vi "CANOpen Addon Initialization VI.vi"(8 "error in (no error)":errorcluster, 10 "Custom XML":string, 11 "Device Item Ref in":T1 format="%.0x") -> (0 "error out":errorcluster, 3 "Device Item Ref out":T1 format="%.0x")   [LabVIEW 2013, in "CANOpen Addon Custom Device.lvlib"]
uses:
  CANOpen Addon Custom Device.lvlib
  <vilib>/NI Veristand/Custom Device API/Custom Device Item Ref.ctl
  <vilib>/NI Veristand/Custom Device API/Custom Device Channel.ctl
  <vilib>/NI Veristand/Custom Device API/Custom Device Channel Type.ctl
  Shared Code/CANOpen Addon GUID Lookup Global.vi
  <vilib>/NI Veristand/Custom Device API/Custom Device API.lvlib
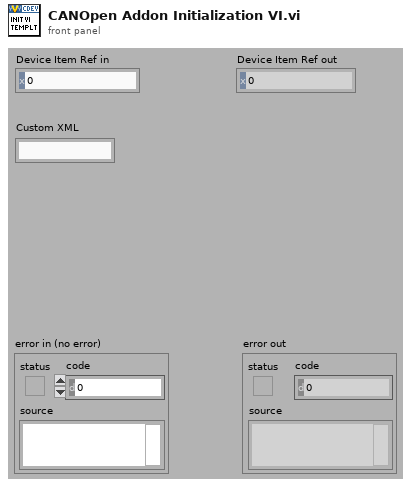
[diagram p1: front panel]
types:
  T1 = typedef "Custom Device API.lvlib/Custom Device Item Ref.ctl" = u64
  T2 = typedef "Custom Device API.lvlib/Custom Device Channel.ctl" = cluster{"Type":T3, "Units":string, "Default Value":dbl, "Faultable":bool, "Scalable":bool}
  T3 = typedef "Custom Device API.lvlib/Custom Device Channel Type.ctl" = enum16{"Input", "Output"}
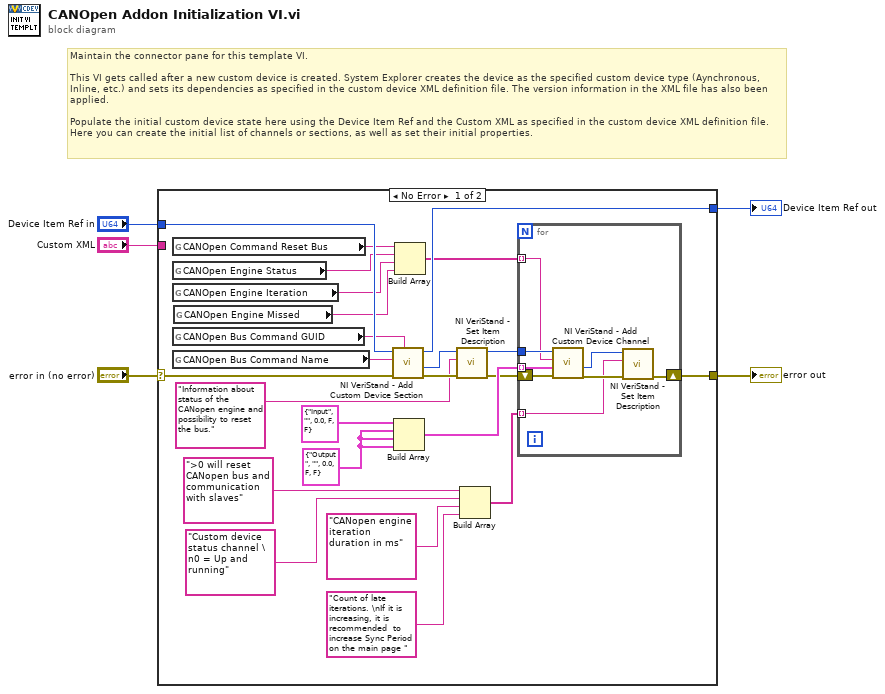
[diagram p0: block diagram]
diagram:
  # "Maintain the connector pane for this template VI.\n\nThis VI gets called after a new custom device is created. System Explorer creates the device as the specified custom device type (Aynchronous, Inline, etc.) and sets its dependencies as specified in the custom device XML definition file. The version information in the XML file has also been applied.\n\nPopulate the initial custom device state here using the Device Item Ref and the Custom XML as specified in the custom device XML definition file. Here you can create the initial list of channels or sections, as well as set their initial properties."
  n1 = case shown="No Error" "error in (no error)" {
    selector: "error in (no error)" -> [w29 w39]
    tunnel: [w28 w39] -> w5
    tunnel: [w26 w38] -> w3
    tunnel: "Device Item Ref in" -> [w27 w38]
    tunnel: "Custom XML" -> [_ _]
    frame No Error {
      w13 = T2 {"Type"=enum."Output", "Units"="", "Default Value"=0.0, "Faultable"=FALSE, "Scalable"=FALSE} ("Channel")
      n2 = global read "CANOpen Addon GUID Lookup Global.vi" "CANOpen Command Reset Bus"() -> (w23:string)
      n3 = global read "CANOpen Addon GUID Lookup Global.vi" "CANOpen Engine Status"() -> (w19:string)
      n4 = global read "CANOpen Addon GUID Lookup Global.vi" "CANOpen Engine Iteration"() -> (w15:string)
      n5 = global read "CANOpen Addon GUID Lookup Global.vi" "CANOpen Bus Command GUID"() -> (w25:string)
      n6 = global read "CANOpen Addon GUID Lookup Global.vi" "CANOpen Bus Command Name"() -> (w24:string)
      n7 = global read "CANOpen Addon GUID Lookup Global.vi" "CANOpen Engine Missed"() -> (w14:string)
      n8 = call <vilib>:"NI VeriStand - Add Custom Device Section.vi"("GUID (Default Section)"=w25, "error in (no error)"=w29, "Section Name"=w24, "Parent Ref in"=w27) -> ("error out"=w10:errorcluster, "Section Ptr"=w8:T1, "Parent Ref out"=w26:T1)  [unwired: 4 in, 1 out]
      n9 = Build Array(T2 {"Type"=enum."Input", "Units"="", "Default Value"=0.0, "Faultable"=FALSE, "Scalable"=FALSE} ("Channel"), w13, w13, w13) -> (w20:T2[])
      n10 = Build Array(w23, w19, w15, w14) -> (w22:string[])
      n11 = call <vilib>:"NI VeriStand - Set Item Description.vi"("error in (no error)"=w10, "Description"="Information about status of the CANopen engine and possibility to reset the bus.", "Item Ref in"=w8) -> ("error out"=w9:errorcluster, "Item Ref out"=w7:T1)  [unwired: 6 in, 1 out]
      n12 = Build Array(">0 will reset CANopen bus and communication with slaves", "Custom device status channel \n0 = Up and running", "CANopen engine iteration duration in ms", "Count of late iterations. \nIf it is increasing, it is recommended  to increase Sync Period on the main page ") -> (w17:string[])
      n13 = for {
        shift-right: [w32] -> w28
        shift-left: w9 -> [w37]
        tunnel: w7 -> [w36]
        tunnel: w22 -> [w35] mode=indexing
        tunnel: w20 -> [w34] mode=indexing
        tunnel: w17 -> [w30] mode=indexing
        n14 = call <vilib>:"NI VeriStand - Add Custom Device Channel.vi"("error in (no error)"=w37, "Channel"=w34, "Channel Name"=w35, "Parent Ref in"=w36) -> ("error out"=w33:errorcluster, "Channel Ref"=w31:T1)  [unwired: 4 in, 2 out]
        n15 = call <vilib>:"NI VeriStand - Set Item Description.vi"("error in (no error)"=w33, "Description"=w30, "Item Ref in"=w31) -> ("error out"=w32:errorcluster)  [unwired: 6 in, 2 out]
      }
    }
    frame Error {
    }
  }
  "error out" <- w5
  "Device Item Ref out" <- w3
